vi "Git-Enterprise-Get All Commits in Repo.vi"(8 "Error In":errorcluster, 9 "Repo":T2={"ID"="1293", "name"="P712-JWA-RCS-CODE1", "full_name"="P887/P712-JWA-RCS-CODE1", "private"="true", "html_url"="https://github.inbcu.com/P887/P712-JWA-RCS-CODE1", "description"="Project 712 RCS 1 Repository", "url"="https://github.inbcu.com/api/v3/repos/P887/P712-JWA-RCS-CODE1"}, 10 "Server":string, 11 "Refnum in":T3) -> (0 "Error out":errorcluster, 3 "Commits":T1[](array[typedef]))   [LabVIEW 2020]
uses:
  <vilib>/httpClient/ClientHandle.ctl
  Git-Repo JSON Typedef.ctl
  Git-Commit JSON Typedef.ctl
  <vilib>/JDP Science/JSONtext/String Subset.vi
  <vilib>/JDP Science/JSONtext/Parsing/Parse Full Path or Item Name.vi
  <vilib>/JDP Science/JSONtext/Offset/Find Item Locations by Path.vi
  <vilib>/httpClient/LabVIEWHTTPClient.lvlib
  <vilib>/JDP Science/JSONtext/JSONtext.lvlib
panel:
  in  "Organization":string
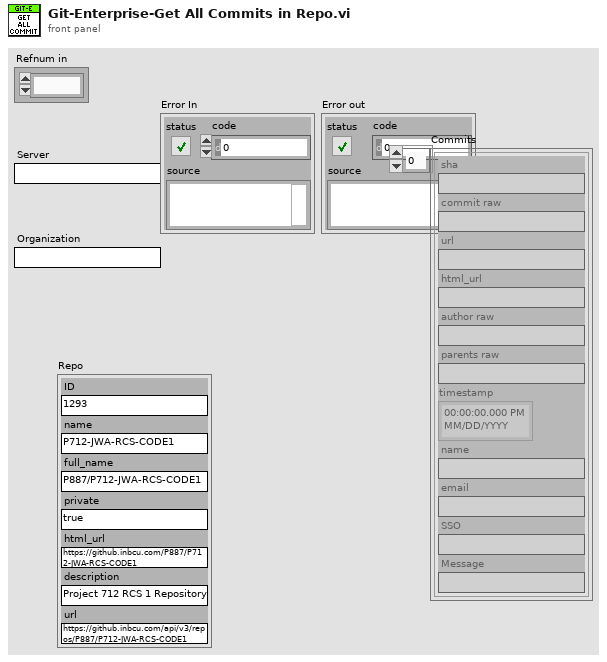
[diagram p1: front panel]
types:
  T1 = typedef "Git-Commit JSON Typedef.ctl" = cluster{"sha":string, "commit raw":string, "url":string, "html_url":string, "author raw":string, "parents raw":string, "timestamp":timestamp, "name":string, "email":string, "SSO":string, "Message":string}
  T2 = typedef "Git-Repo JSON Typedef.ctl" = cluster{"ID":string, "name":string, "full_name":string, "private":string, "html_url":string, "description":string, "url":string}
  T3 = typedef "LabVIEWHTTPClient.lvlib/ClientHandle.ctl" = refnum<k1>
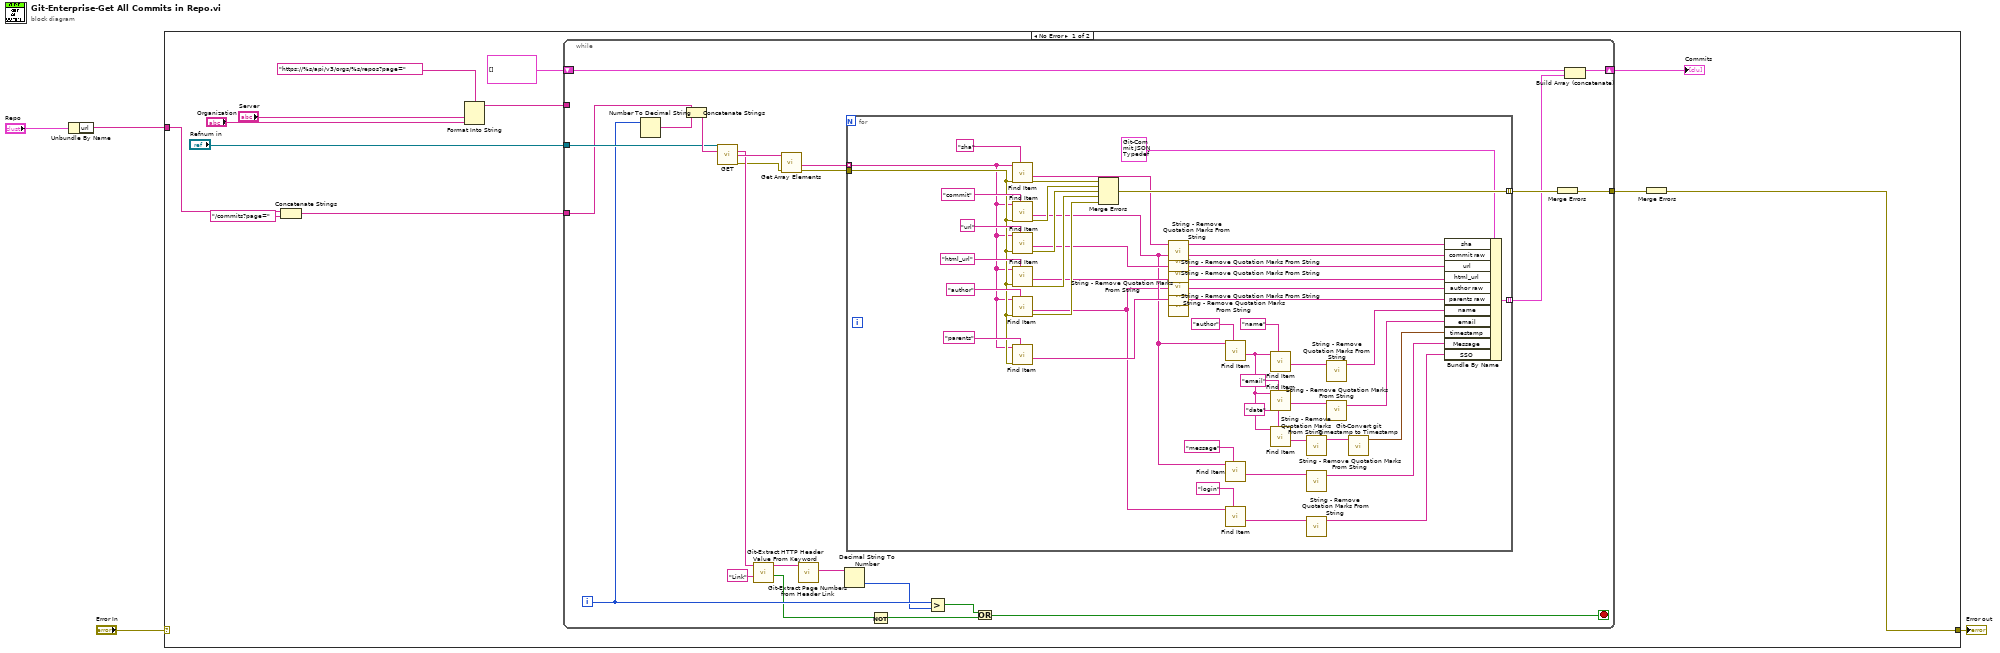
[diagram p0: block diagram]
diagram:
  n1 = Unbundle By Name("Repo") -> ("url"=w1:string)
  n2 = case shown="No Error" "Error In" {
    selector: "Error In" -> [_ w86]
    tunnel: [w9 w86] -> w3
    tunnel: w1 -> [w8 _]
    frame No Error {
      n3 = Concatenate Strings(w8, "/commits?page=" ("string")) -> (w6:string)
      n4 = Format Into String(format string="https://%s/api/v3/orgs/%s/repos?page=" ("url"), "Server", "Organization") -> (resulting string=w16:string)  [unwired: 2 in, 1 out]
      n5 = while {
        tunnel: "Refnum in" -> [w38]
        shift-right: [w34] -> w5
        shift-left: T1[] [] -> [w35]
        tunnel: w16 -> [_]
        tunnel: [w24] -> w10
        tunnel: w6 -> [w17]
        i -> [w37]
        stop <- w19 stop-if-true
        n6 = Number To Decimal String(number=w37) -> (decimal integer string=w36:string)  [unwired: 1 in]
        n7 = Concatenate Strings(w17, w36) -> (w39:string)
        n8 = call <vilib>:"GET.vi"("client handle"=w38, "url"=w39) -> ("headers"=w27:string, "body"=w31:string, "error out"=w23:errorcluster)  [unwired: 10 in, 1 out]
        n9 = call "Git-Extract HTTP Header Value From Keyword.vi"("Key"="Link", "Header Info"=w27) -> ("Found"=w21:bool, "Value"=w28:string)  [unwired: 8 in]
        n10 = call <vilib>:"Get Array Elements.vi"("error in (no error)"=w23, "JSON"=w31) -> ("error out"=w33:errorcluster, "<JSON>"=w32:string[])  [unwired: 7 in, 1 out]
        n11 = call "Git-Extract Page Numbers from Header Link.vi"("Link"=w28) -> ("Pages"=w30:string)  [unwired: 9 in, 1 out]
        n12 = Decimal String To Number(string=w30) -> (number=w26:i32)  [unwired: 2 in, 1 out]
        n13 = for {
          tunnel: w32 -> [w71] mode=indexing
          tunnel: w33 -> [w72]
          tunnel: [w75] -> w25 mode=indexing
          tunnel: [w73] -> w18 mode=indexing
          n14 = call <vilib>:"Find Item.vi"("$Path or Item Name"="commit", "error in (no error)"=w72, "JSON"=w71) -> ("error out"=w79:errorcluster, "<JSON>"=w47:string)  [unwired: 5 in, 2 out]
          n15 = call <vilib>:"Find Item.vi"("$Path or Item Name"="url", "error in (no error)"=w72, "JSON"=w71) -> ("error out"=w78:errorcluster, "<JSON>"=w68:string)  [unwired: 5 in, 2 out]
          n16 = call <vilib>:"Find Item.vi"("$Path or Item Name"="html_url", "error in (no error)"=w72, "JSON"=w71) -> ("error out"=w77:errorcluster, "<JSON>"=w66:string)  [unwired: 5 in, 2 out]
          n17 = call <vilib>:"Find Item.vi"("$Path or Item Name"="author", "error in (no error)"=w72, "JSON"=w71) -> ("error out"=w76:errorcluster, "<JSON>"=w43:string)  [unwired: 5 in, 2 out]
          n18 = call <vilib>:"Find Item.vi"("$Path or Item Name"="parents", "error in (no error)"=w72, "JSON"=w71) -> ("<JSON>"=w63:string)  [unwired: 5 in, 3 out]
          n19 = call <vilib>:"Find Item.vi"("$Path or Item Name"="sha", "error in (no error)"=w72, "JSON"=w71) -> ("error out"=w80:errorcluster, "<JSON>"=w70:string)  [unwired: 5 in, 2 out]
          n20 = Merge Errors(w80, w79, w78, w77, w76) -> (w75:errorcluster)
          n21 = call "String - Remove Quotation Marks From String.vi"("String"=w70) -> ("result string"=w69:string)  [unwired: 4 in]
          n22 = call "String - Remove Quotation Marks From String.vi"("String"=w47) -> ("result string"=w60:string)  [unwired: 4 in]
          n23 = call "String - Remove Quotation Marks From String.vi"("String"=w68) -> ("result string"=w67:string)  [unwired: 4 in]
          n24 = call "String - Remove Quotation Marks From String.vi"("String"=w66) -> ("result string"=w65:string)  [unwired: 4 in]
          n25 = call "String - Remove Quotation Marks From String.vi"("String"=w43) -> ("result string"=w64:string)  [unwired: 4 in]
          n26 = call "String - Remove Quotation Marks From String.vi"("String"=w63) -> ("result string"=w62:string)  [unwired: 4 in]
          n27 = call <vilib>:"Find Item.vi"("$Path or Item Name"="author", "JSON"=w47) -> ("<JSON>"=w54:string)  [unwired: 6 in, 3 out]
          n28 = call <vilib>:"Find Item.vi"("$Path or Item Name"="message", "JSON"=w47) -> ("<JSON>"=w45:string)  [unwired: 6 in, 3 out]
          n29 = call <vilib>:"Find Item.vi"("$Path or Item Name"="login", "JSON"=w43) -> ("<JSON>"=w41:string)  [unwired: 6 in, 3 out]
          n30 = call <vilib>:"Find Item.vi"("$Path or Item Name"="name", "JSON"=w54) -> ("<JSON>"=w57:string)  [unwired: 6 in, 3 out]
          n31 = call <vilib>:"Find Item.vi"("$Path or Item Name"="email", "JSON"=w54) -> ("<JSON>"=w52:string)  [unwired: 6 in, 3 out]
          n32 = call <vilib>:"Find Item.vi"("$Path or Item Name"="date", "JSON"=w54) -> ("<JSON>"=w50:string)  [unwired: 6 in, 3 out]
          n33 = call "String - Remove Quotation Marks From String.vi"("String"=w50) -> ("result string"=w49:string)  [unwired: 4 in]
          n34 = call "String - Remove Quotation Marks From String.vi"("String"=w45) -> ("result string"=w44:string)  [unwired: 4 in]
          n35 = call "String - Remove Quotation Marks From String.vi"("String"=w41) -> ("result string"=w40:string)  [unwired: 4 in]
          n36 = call "String - Remove Quotation Marks From String.vi"("String"=w57) -> ("result string"=w56:string)  [unwired: 4 in]
          n37 = call "String - Remove Quotation Marks From String.vi"("String"=w52) -> ("result string"=w51:string)  [unwired: 4 in]
          n38 = call "Git-Convert git Timestamp to Timestamp.vi"("Git Timestamp"=w49) -> ("Time Stamp"=w48:timestamp)  [unwired: 4 in]
          n39 = Bundle By Name(cluster=T1 {"sha"="", "commit raw"="", "url"="", "html_url"="", "author raw"="", "parents raw"="", "timestamp"=timestamp(0 s since 1904-01-01), "name"="", "email"="", "SSO"="", "Message"=""}, "sha"=w69, "commit raw"=w60, "url"=w67, "html_url"=w65, "author raw"=w64, "parents raw"=w62, "name"=w56, "email"=w51, "timestamp"=w48, "Message"=w44, "SSO"=w40) -> (w73:T1)
        }
        n40 = Not(x=w21) -> (.not. x?=w22:bool)
        n41 = Greater?(x=w37, y=w26) -> (0:w20:bool)
        n42 = Or(x=w20, y=w22) -> (x .or. y?=w19:bool)
        n43 = Merge Errors(w25) -> (w24:errorcluster)
        n44 = Build Array (concatenate)(w35, w18) -> (w34:T1[])
      }
      "Commits" <- w5
      n45 = Merge Errors(w10) -> (w9:errorcluster)
    }
    frame Error {
    }
  }
  "Error out" <- w3
